vi "PH_Beckhoff_PP_PU.declare analog OutputTags.vi"(3 "PU Type":T4) -> (0 "Analog Outputs":T3, 1 "Description":string)   [LabVIEW 2014, in "PH_Beckhoff_PP_PU.lvlib"]
uses:
  PH_Beckhoff_PP_PU.lvlib
  PH_Beckhoff_PP_PU.PU Rack Type.ctl
  PH_Beckhoff/PH_Beckhoff.Analog Outputs.ctl
  PH_Beckhoff/PH_Beckhoff.Scaling Type.ctl
  PH_PP_Common/PH_PP_Common.PSU Tags.ctl
  PH_Beckhoff/PH_Beckhoff.lvlib
  PH_PP_Common/PH_PP_Common.lvlib
panel:
  in  "Analog Output Value":T2
  out "Right Size?":bool
  # "Let this VI run to check the size!"
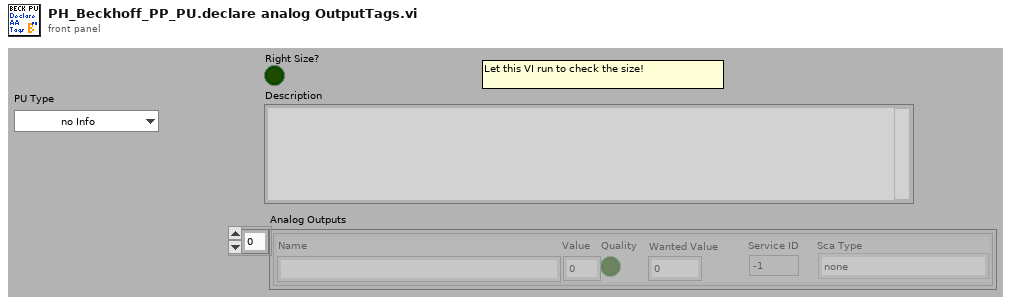
[diagram p1: front panel]
types:
  T1 = typedef "PH_Beckhoff.lvlib/PH_Beckhoff.Scaling Type.ctl" = enum16{"none", "0 ... 15 Bit -> 0 ... 5", "0 ... 15 Bit -> 0 ... 10", "0 ... 15 Bit -> 0 ... 25", "0 ... 15 Bit -> 4 ... 20", "0 ... 15 Bit -> 0 ... 1", "0 ... 15 Bit -> 0 ... 20000", "0 ... 15 Bit -> 0 ... 24000"}
  T2 = cluster{"Name":string, "Value":u32, "Quality":bool, "Wanted Value":u32, "Service ID":i32, "Sca Type":T1}
  T3 = typedef "PH_Beckhoff.lvlib/PH_Beckhoff.Analog Outputs.ctl" = cluster{"Name":string, "Value":u32, "Quality":bool, "Wanted Value":u32, "Service ID":i32, "Sca Type":T1}[]
  T4 = typedef "PH_Beckhoff_PP_PU.lvlib/PH_Beckhoff_PP_PU.PU Rack Type.ctl" = enum16{"no Info", "PA 19mm", "PA 45mm", "MA PU 1 and 2", "MA PU 3 and 4", "MA PU 5 and 6", "MA FR and PILC"}
  T5 = typedef "PH_PP_Common.lvlib/PH_PP_Common.PSU Tags.ctl" = enum16{"voltage-indicator", "peak-detect", "current", "voltage", "inihibit-indicator", "end-of-charge", "HV-on-indicator", "overtemperature", "interlock-indicator", "load-fault", "sum-fault", "HV-off-indicator", "DC-ok", "inhibit", "HV-on", "interlock", "reset", "Status", "Limits"}
  T6 = typedef "PH_PP_Common.lvlib/PH_PP_Common.PUs.ctl" = enum16{"no Info", "PA-19mm-1", "PA-19mm-2", "PA-45mm-PILC", "PA-45mm-MAIN", "MA-PU-1", "MA-PU-2", "MA-PU-3", "MA-PU-4", "MA-PU-5", "MA-PU-6", "MA-FR", "MA-PILC", "PA-45mm-DP"}
  T7 = typedef "PH_PP_Common.lvlib/PH_PP_Common.PSU Type.ctl" = enum16{"none", "Maxwell Standard", "DEL", "Maxwell ALE", "Continuum 601k"}
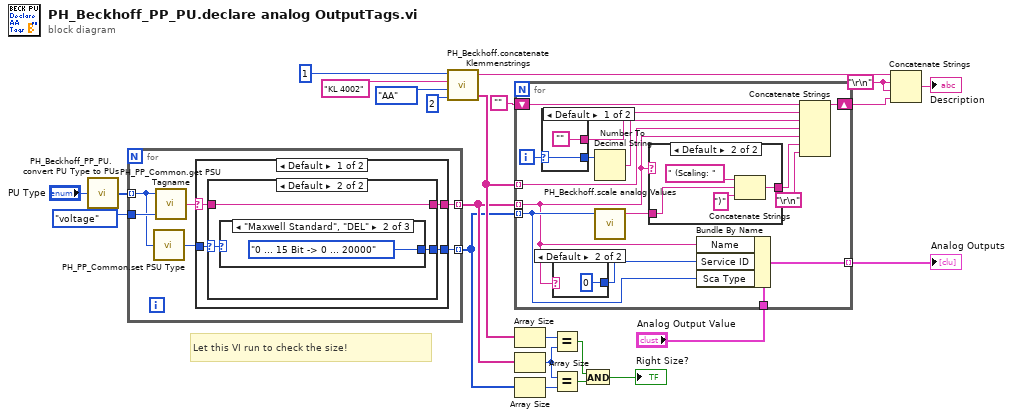
[diagram p0: block diagram]
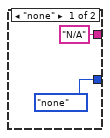
[diagram p2: hidden frame]
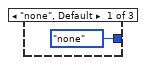
[diagram p3: hidden frame]
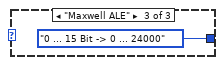
[diagram p4: hidden frame]
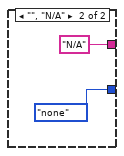
[diagram p5: hidden frame]
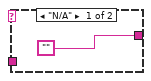
[diagram p6: hidden frame]
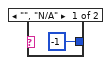
[diagram p7: hidden frame]
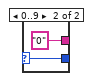
[diagram p8: hidden frame]
diagram:
  w21 = "\r\n"
  # "Let this VI run to check the size!"
  n1 = call "PH_Beckhoff_PP_PU.convert PU Type to PUs.vi"("PU Type"="PU Type") -> ("PUs"=w3:T6[])
  n2 = for {
    tunnel: [w29] -> w6 mode=indexing
    tunnel: [w28] -> w5 mode=indexing
    tunnel: w3 -> [w24] mode=indexing
    tunnel: PH_PP_Common.PSU_Tags."voltage" ("PSU Tag") -> [w26]
    n3 = call "PH_PP_Common.set PSU Type.vi"("PU"=w24) -> ("PSU Type"=w25:T7)
    n4 = call "PH_PP_Common.get PSU Tagname.vi"("PSU Tag"=w26, "PU"=w24) -> ("PSU Tagname"=w27:string)  [unwired: 1 in]
    n5 = case shown="Default" w27 {
      selector: w27 -> [w33 _]
      tunnel: [w32 "N/A"] -> w29
      tunnel: [w30 PH_Beckhoff.Scaling_Type."none" ("Sca Type")] -> w28
      tunnel: w25 -> [w31 _]
      frame Default {
        n6 = case shown="Default" w31 {
          selector: w31 -> [_ w38]
          tunnel: w33 -> [_ w36]
          tunnel: ["N/A" w36] -> w32
          tunnel: [PH_Beckhoff.Scaling_Type."none" ("Sca Type") w37] -> w30
          frame "none" {
          }
          frame Default {
            n7 = case shown="\"Maxwell Standard\", \"DEL\"" w38 {
              tunnel: [PH_Beckhoff.Scaling_Type."none" ("Sca Type") PH_Beckhoff.Scaling_Type."0 ... 15 Bit -> 0 ... 20000" ("Sca Type") PH_Beckhoff.Scaling_Type."0 ... 15 Bit -> 0 ... 24000" ("Sca Type")] -> w37
              frame "none", Default {
              }
              frame "Maxwell Standard", "DEL" {
              }
              frame "Maxwell ALE" {
              }
            }
          }
        }
      }
      frame "", "N/A" {
      }
    }
  }
  n8 = call "PH_Beckhoff.concatenate Klemmenstrings.vi"("# of In- or Outputs"=2, "Type"=enum16{"AE", "AA", "DE", "DA", "SE"}."AA", "Klemmenname"="KL 4002", "Quantity"=1) -> ("concatenated string array"=w9:string[], "\"<Type>: <Quantity> x <Klemmenname>\""=w10:string)  [unwired: 1 out]
  n9 = for {
    tunnel: w6 -> [w44] mode=indexing
    tunnel: w9 -> [w54] mode=indexing
    shift-right: [w46] -> w22
    shift-left: "" -> [w47]
    tunnel: w5 -> [w50] mode=indexing
    tunnel: "Analog Output Value" -> [w49]
    tunnel: [w51] -> w7 mode=indexing
    i -> [w58]
    n10 = case shown="Default" w58 {
      selector: w58 -> [w66 w69]
      tunnel: [w66 w69] -> w57
      tunnel: ["" "0"] -> w56
      frame Default {
      }
      frame 0..9 {
      }
    }
    n11 = case shown="Default" w44 {
      tunnel: [-1 ("Service ID") 0 ("Service ID")] -> w52
      frame "", "N/A" {
      }
      frame Default {
      }
    }
    n12 = Number To Decimal String(number=w57) -> (decimal integer string=w55:string)  [unwired: 1 in]
    n13 = call "PH_Beckhoff.scale analog Values.vi"("Sca Type"=w50) -> ("Scaling"=w48:string)  [unwired: 2 in, 2 out]
    n14 = case shown="Default" w44 {
      tunnel: ["" w62] -> w53
      tunnel: w48 -> [_ w61]
      frame "N/A" {
      }
      frame Default {
        n15 = Concatenate Strings(" (Scaling: " ("string"), w61, ")" ("string")) -> (w62:string)
      }
    }
    n16 = Bundle By Name(cluster=w49, "Name"=w44, "Service ID"=w52, "Sca Type"=w50) -> (w51:T2)
    n17 = Concatenate Strings(w47, w56, w55, w54, w44, w53, "\r\n") -> (w46:string)
  }
  "Analog Outputs" <- w7
  n18 = Array Size(array=w9) -> (size(s)=w19:i32)
  n19 = Array Size(array=w6) -> (size(s)=w15:i32)
  n20 = Array Size(array=w5) -> (size(s)=w14:i32)
  n21 = Equal?(x=w19, y=w15) -> (x = y?=w18:bool)
  n22 = Equal?(x=w15, y=w14) -> (x = y?=w12:bool)
  n23 = And(x=w18, y=w12) -> (x .and. y?=→"Right Size?":bool)
  n24 = Concatenate Strings(w10, w21, w21, w22) -> (→"Description":string)
